vi "Dequeue And Send Value.vi"(0 "VI reference":refnum<vi>, 1 "queue in":refnum<queue>, 2 "error in":errorcluster) -> (3 "dup VI Refnum":refnum<vi>, 4 "queue out":refnum<queue>, 5 "Queue Err":bool, 6 "error out":errorcluster)   [LabVIEW 2020]
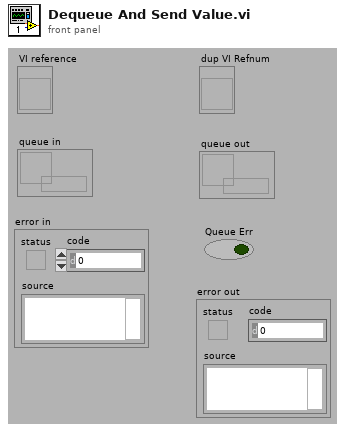
[diagram p1: front panel]
types:
  T1 = enum32{"Bad", "Idle", "Run top level", "Running"}
  T2 = cluster{"Control Name":string, "Type Descriptor":i16[], "Flattened Data":string}
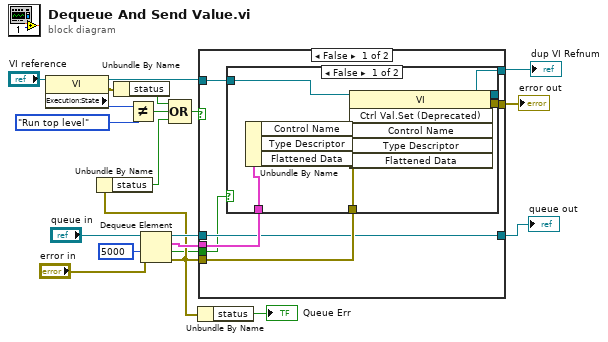
[diagram p0: block diagram]
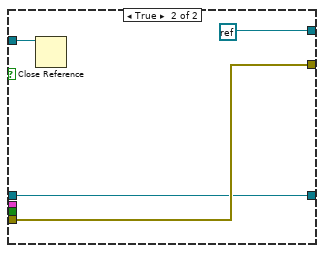
[diagram p3: hidden frame]
diagram:
  n1 = property class="VI"(reference="VI reference") -> (reference out=w17:refnum<vi>, error out=w12:errorcluster, "Execution:State"=w16:T1)  [unwired: 1 in]
  n2 = Unbundle By Name(w12) -> ("status"=w11:bool)
  n3 = Not Equal?(x=w16, y=T1."Run top level" ("Execution:State")) -> (x != y?=w14:bool)
  n4 = Dequeue Element(queue="queue in", timeout in ms (-1)=5000, error in (no error)="error in") -> (queue out=w5:refnum<queue>, element=w10:T2, timed out?=w1:bool, error out=w4:errorcluster)
  n5 = Unbundle By Name(w4) -> ("status"=w9:bool)
  n6 = Compound Arithmetic op=OR(w11, w14, w9) -> (w13:bool)
  n7 = Unbundle By Name(w4) -> ("status"=→"Queue Err":bool)
  n8 = case shown="False" w13 {
    tunnel: [w27 refnum<k0> refnum ("Not a Refnum Constant")] -> w20
    tunnel: [w26 w41] -> w19
    tunnel: w4 -> [w24 w41]
    tunnel: w5 -> [w22 w38]
    tunnel: w17 -> [w25 w40]
    tunnel: w10 -> [w23 _]
    tunnel: [w22 w38] -> w8
    tunnel: w1 -> [w21 _]
    frame False {
      n9 = case shown="False" w21 {
        tunnel: [w35 w37] -> w27
        tunnel: [w34 w36] -> w26
        tunnel: w25 -> [w30 w37]
        tunnel: w24 -> [w29 w36]
        tunnel: w23 -> [w28 _]
        frame False {
          n10 = Unbundle By Name(w28) -> ("Control Name"=w33:string, "Type Descriptor"=w31:i16[], "Flattened Data"=w32:string)
          n11 = invoke class="VI" method="Ctrl Val.Set (Deprecated)"(reference=w30, error in=w29, "Control Name"=w33, "Type Descriptor"=w31, "Flattened Data"=w32) -> (reference out=w35:refnum<vi>, error out=w34:errorcluster)  [unwired: 1 in, 4 out]
        }
        frame True {
        }
      }
    }
    frame True {
      n12 = Close Reference(reference=w40) -> ()  [unwired: 1 in, 1 out]
    }
  }
  "dup VI Refnum" <- w20
  "error out" <- w19
  "queue out" <- w8
